vi "Call Measure tool.vi"(8 "error in (no error)":errorcluster, 11 "Path":path) -> (0 "error out":errorcluster)   [LabVIEW 2020]
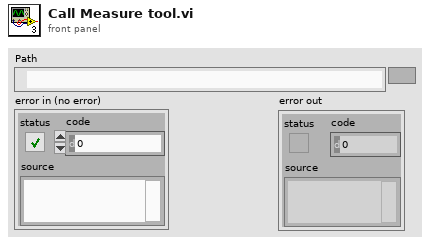
[diagram p1: front panel]
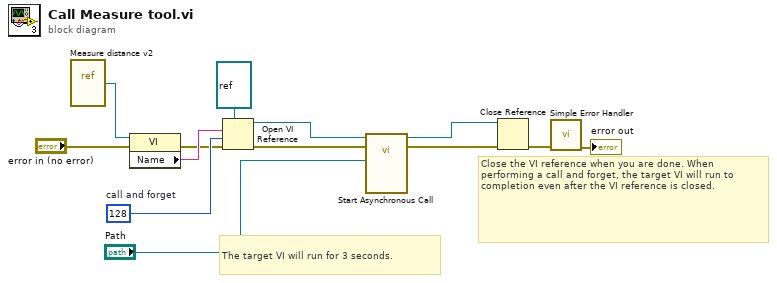
[diagram p0: block diagram]
diagram:
  w13 = 128  # call and forget
  # "Close the VI reference when you are done. When performing a call and forget, the target VI will run to completion even after the VI reference is closed."
  # "The target VI will run for 3 seconds."
  n1 = vi-ref "Measure distance v2.vi"() -> (w6:refnum<vi>)
  n2 = property class="VI"(reference=w6, error in="error in (no error)") -> (error out=w4:errorcluster, "Name"=w5:string)  [unwired: 1 out]
  n3 = Open VI Reference(type specifier VI Refnum (for type only)=refnum<vi> refnum, vi path=w5, options=w13, error in (no error)=w4) -> (vi reference=w11:refnum<vi>, error out=w10:errorcluster)  [unwired: 2 in]
  n4 = call-by-ref "Start Asynchronous Call"(reference=w11, error in=w10, "Path"="Path") -> (reference out=w8:refnum<vi>, error out=w9:errorcluster)  [unwired: 10 in, 1 out]
  n5 = Close Reference(reference=w8, error in (no error)=w9) -> (error out=w7:errorcluster)
  n6 = call <vilib>:"Simple Error Handler.vi"("error in (no error)"=w7) -> ("error out"=→"error out":errorcluster)  [unwired: 4 in, 4 out]
